vi "Open.vi"(8 "error in (no error)":errorcluster, 11 "MelsecTCP in":refnum<class "InovanceModbusTcp.lvclass">) -> (0 "error out":errorcluster, 3 "MelsecTCP out":refnum<class "InovanceModbusTcp.lvclass">)   [LabVIEW 2020, in "HslCommunication.lvlib" / "InovanceModbusTcp.lvclass"]
uses:
  InovanceModbusTcp.lvclass
  D:/Project/Labview-Projects/General utility tool/Libraries/HslCommunication/Abstract PLC Controler/Abstract PLC Controler.lvclass
  EventLogger.lvlibp/1abvi3w/vi.lib/gpm_packages/@cs/event-logger/Source/Composed Log/Types/Log Level.ctl
  Abstract PLC Controler/Abstract PLC Controler.lvclass/Abstract PLC Controler.ctl
  InovanceModbusTcp.lvclass/InovanceModbusTcp.ctl
  D:/Project/Labview-Projects/General utility tool/Libraries/HslCommunication/_Dependenciecs/HslCommunication.dll
  _Dependenciecs/HslCommunication.dll
  Read series.vi
  Read ipAddress.vi
  Read port.vi
  Abstract PLC Controler/Abstract PLC Controler.lvclass
  EventLogger.lvlibp/Logger.lvclass
  EventLogger.lvlibp/1abvi3w/vi.lib/gpm_packages/@cs/event-logger/Source/Composed Log/Composed Log.lvlib
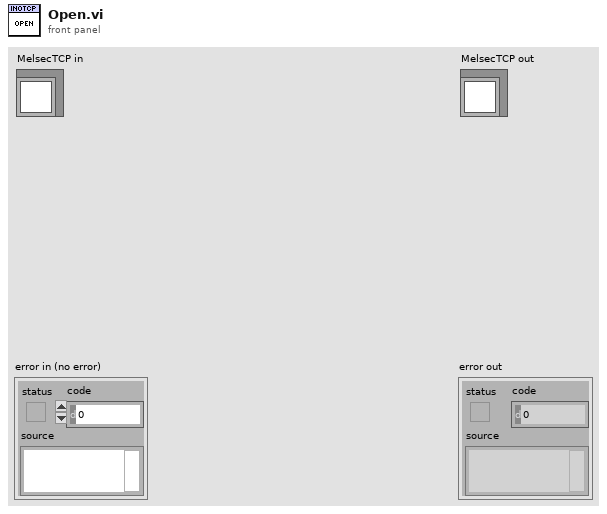
[diagram p1: front panel]
types:
  T1 = typedef "EventLogger.lvlibp/Composed Log.lvlib/Log Level.ctl" = enum16{"Debug", "Info", "Warning", "Error", "Critical"}
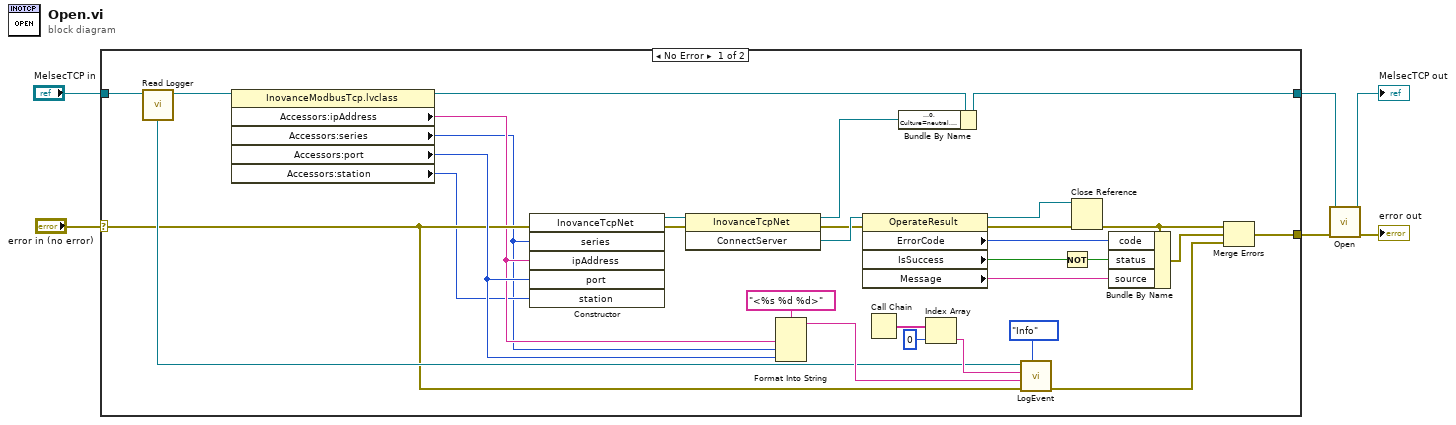
[diagram p0: block diagram]
diagram:
  n1 = case shown="No Error" "error in (no error)" {
    selector: "error in (no error)" -> [w12 w39]
    tunnel: "MelsecTCP in" -> [w37 w38]
    tunnel: [w36 w38] -> w2
    tunnel: [w30 w39] -> w4
    frame No Error {
      n2 = call "Read Logger.vi"("Abstract PLC Controler in"=w37) -> ("EventLogger.lvlibp:Logger.lvclass"=w13:refnum<class "Logger.lvclass">, "Abstract PLC Controler out"=w20:refnum<class "InovanceModbusTcp.lvclass">)  [unwired: 9 in]
      n3 = property class="InovanceModbusTcp.lvclass"(reference=w20) -> (reference out=w21:refnum<class "InovanceModbusTcp.lvclass">, "Accessors:ipAddress"=w9:string, "Accessors:series"=w7:i32, "Accessors:port"=w17:i32, "Accessors:station"=w8:u8)  [unwired: 1 in, 1 out]
      n4 = constructor class="InovanceTcpNet"(error in=w12, "series"=w7, "ipAddress"=w9, "port"=w17, "station"=w8) -> (reference out=w25:refnum<k24>, error out=w24:errorcluster)  [unwired: 2 in, 5 out]
      n5 = invoke class="InovanceTcpNet" method="ConnectServer"(reference=w25, error in=w24) -> (reference out=w22:refnum<k24>, error out=w27:errorcluster, "ConnectServer"=w29:refnum<k24>)  [unwired: 1 in]
      n6 = Format Into String(format string="<%s %d %d>", w9, w7, w17) -> (resulting string=w15:string)  [unwired: 2 in, 1 out]
      n7 = property class="OperateResult"(reference=w29, error in=w27) -> (reference out=w28:refnum<k24>, error out=w26:errorcluster, "ErrorCode"=w33:i32, "IsSuccess"=w23:bool, "Message"=w31:string)
      n8 = Call Chain() -> (call chain=w19:string[])
      n9 = Bundle By Name(cluster=w21, "reference"=w22) -> (w36:refnum<class "InovanceModbusTcp.lvclass">)
      n10 = Index Array(array=w19, index=0) -> (element=w14:string)
      n11 = call "LogEvent.vi"("Event Level"=Log_Level."Info", "error in (no error)"=w12, "Data To Log"=w15, "SourceID"=w14, "Logger in"=w13) -> ("error out"=w11:errorcluster)  [unwired: 5 in, 1 out]
      n12 = Not(x=w23) -> (.not. x?=w32:bool)
      n13 = Close Reference(reference=w28, error in (no error)=w26) -> (error out=w34:errorcluster)
      n14 = Bundle By Name(cluster=w34, "code"=w33, "status"=w32, "source"=w31) -> (w35:errorcluster)
      n15 = Merge Errors(w34, w35, w11) -> (w30:errorcluster)
    }
    frame Error {
    }
  }
  n16 = call-parent "Open.vi"("error in (no error)"=w4, "MelsecTCP in"=w2) -> ("error out"=→"error out":errorcluster, "MelsecTCP out"=→"MelsecTCP out":refnum<class "InovanceModbusTcp.lvclass">)  [unwired: 8 in]
